vi "MCListManager.vi"(8 "error in (no error)":errorcluster, 9 "Path":path, 10 "Command":T1(ring), 11 "MCListbox Refnum":refnum<vi>) -> (0 "error out":errorcluster, 3 "MCListbox Refnum out":refnum<vi>)   [LabVIEW 2013, in "AnimatorXControl.xctl"]
uses:
  AnimatorXControl.xctl
panel:
  out "TempString":string
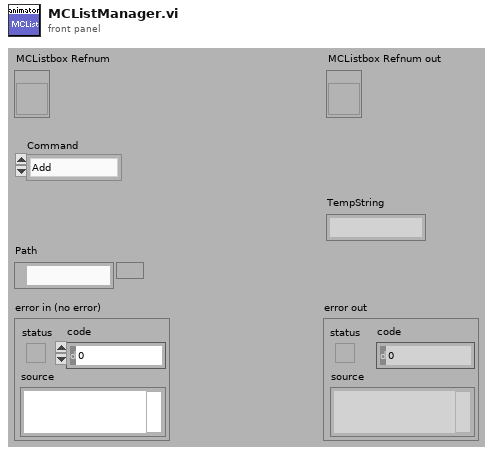
[diagram p1: front panel]
types:
  T1 = enum16{"Add", "Remove", "RemoveAll", "MoveUp", "MoveDown"}
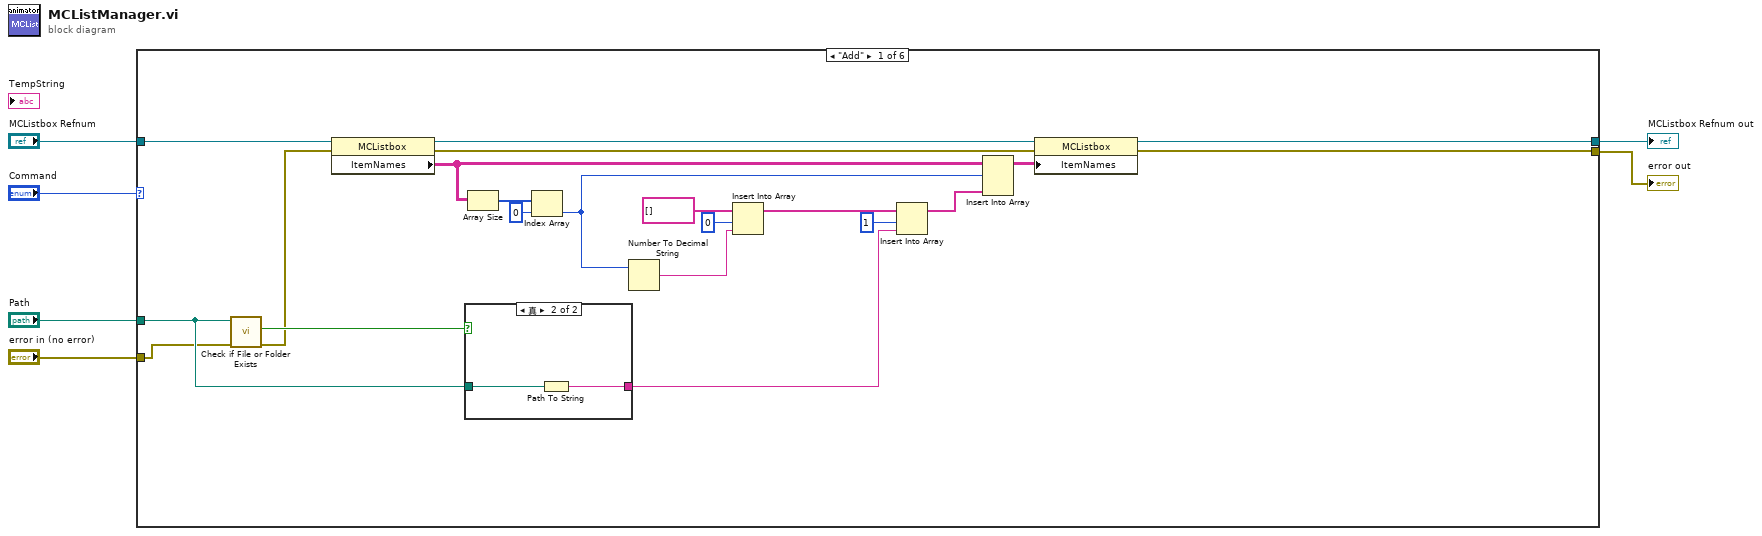
[diagram p0: block diagram]
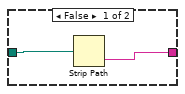
[diagram p2: hidden frame]
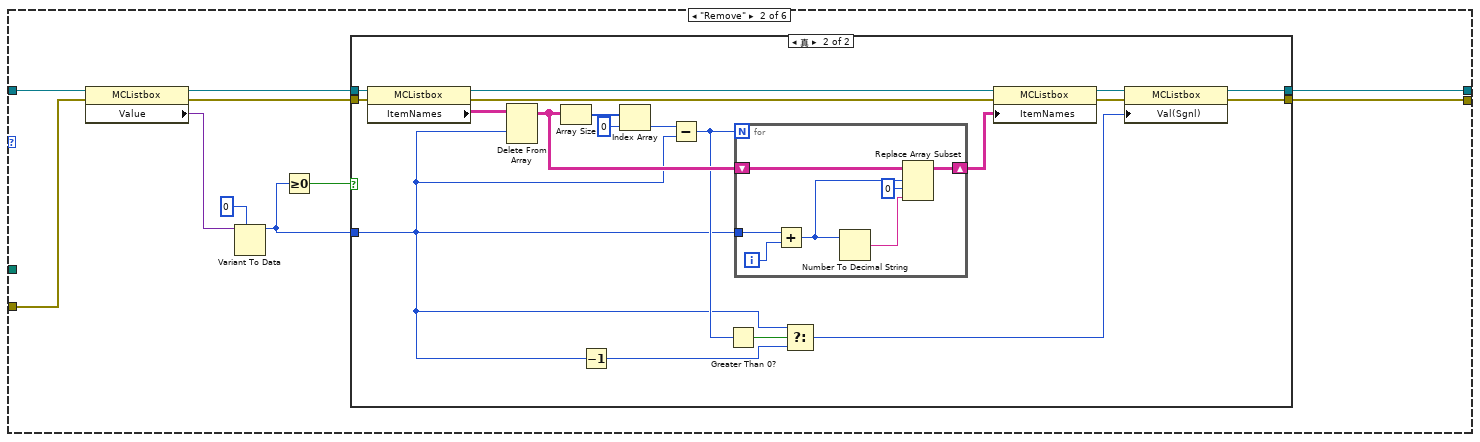
[diagram p3: hidden frame]
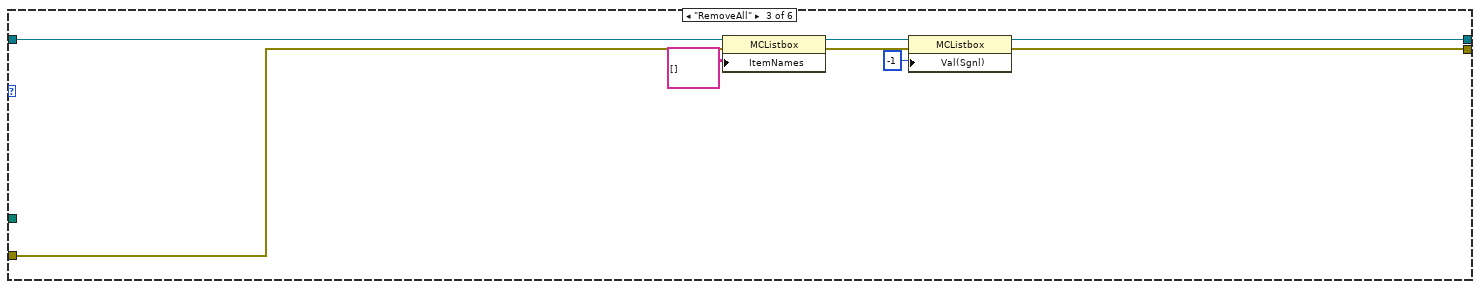
[diagram p5: hidden frame]
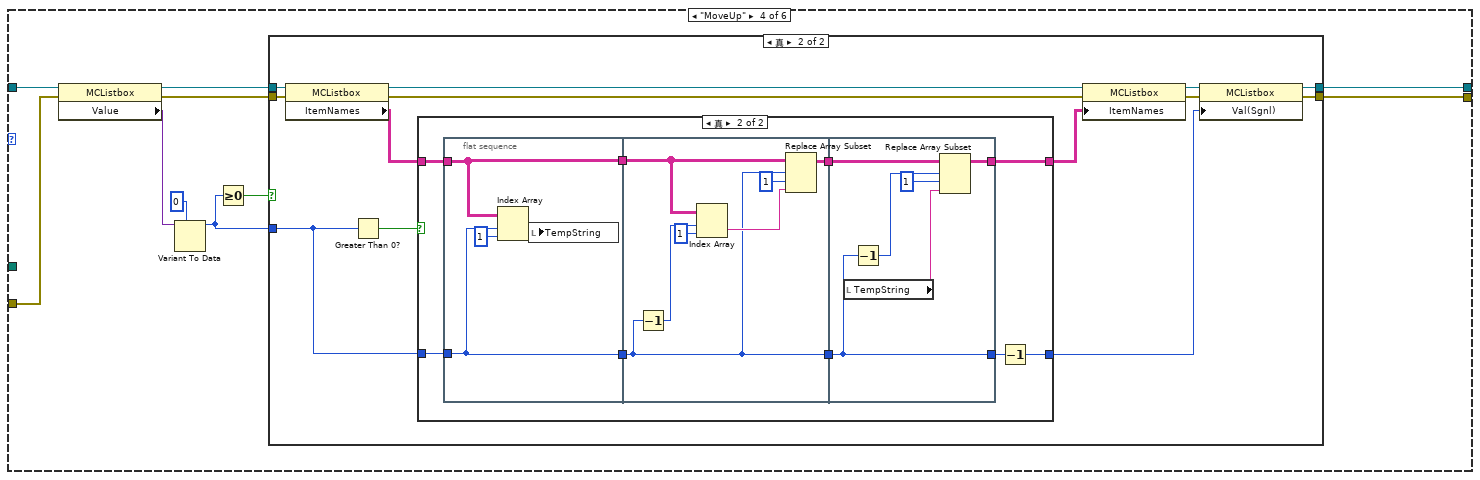
[diagram p6: hidden frame]
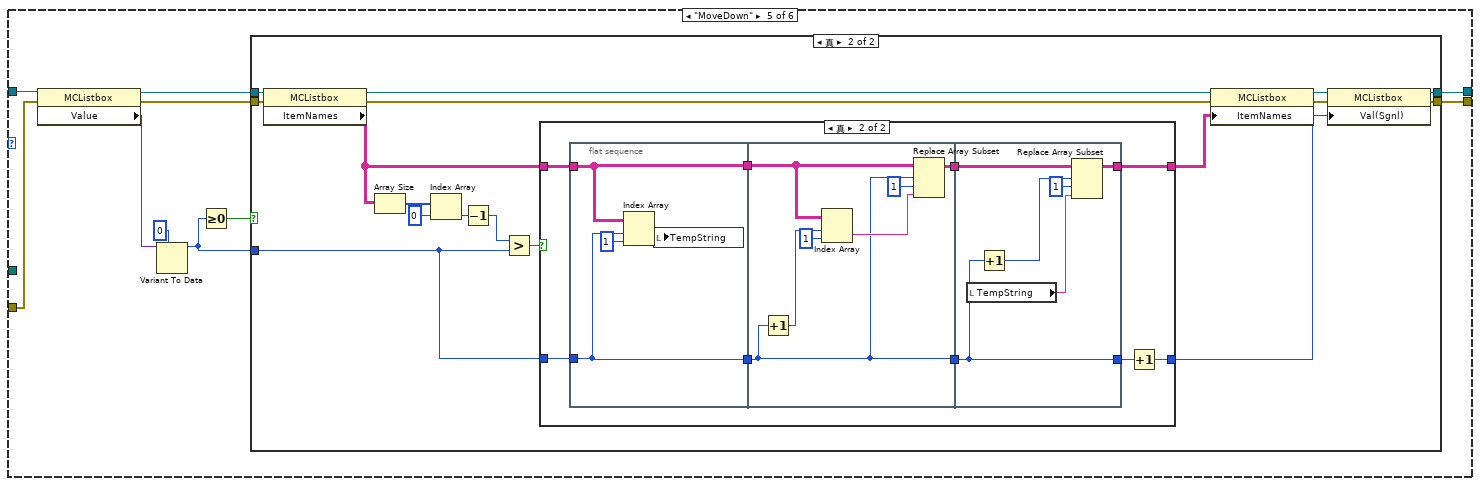
[diagram p9: hidden frame]
diagram:
  n1 = case shown="\"Add\"" "Command" {
    tunnel: "MCListbox Refnum" -> [w20 w36 w72 w87 w138 w188]
    tunnel: "Path" -> [w14 _ _ _ _ _]
    tunnel: [w9 w38 w73 w83 w137 w189] -> w3
    tunnel: "error in (no error)" -> [w11 w39 w71 w84 w136 w189]
    tunnel: [w8 w37 w74 w82 w135 w188] -> w1
    frame "Add" {
      n2 = call <vilib>:"Check if File or Folder Exists.vi"("error in (no error)"=w11, "path"=w14) -> ("error out"=w10:errorcluster, "file or folder exists?"=w15:bool)  [unwired: 7 in, 1 out]
      n3 = property class="MCListbox"(reference=w20, error in=w10) -> (reference out=w19:refnum<vi>, error out=w12:errorcluster, "ItemNames"=w22:string[][])
      n4 = case shown="真" w15 {
        tunnel: w14 -> [w29 w31]
        tunnel: [w28 w30] -> w13
        frame False {
          n5 = Strip Path(path=w29) -> (name=w28:string)  [unwired: 1 out]
        }
        frame True {
          n6 = Path To String(path=w31) -> (string=w30:string)
        }
      }
      n7 = Array Size(array=w22) -> (size(s)=w27:i32[])
      n8 = Index Array(array=w27, index=0) -> (element=w16:i32)
      n9 = Number To Decimal String(number=w16) -> (decimal integer string=w17:string)  [unwired: 1 in]
      n10 = Insert Into Array(array=string[] [], index=0 ("disabled index (col)"), new element=w17) -> (w7:string[])
      n11 = Insert Into Array(array=w7, index=1 ("disabled index (col)"), new element=w13) -> (w21:string[])
      n12 = Insert Into Array(array=w22, index (row)=w16, new element=w21) -> (w18:string[][])  [unwired: 1 in]
      n13 = property class="MCListbox"(reference=w19, error in=w12, "ItemNames"=w18) -> (reference out=w8:refnum<vi>, error out=w9:errorcluster)
    }
    frame "Remove" {
      n14 = property class="MCListbox"(reference=w36, error in=w39) -> (reference out=w41:refnum<vi>, error out=w40:errorcluster, "Value"=w35:variant)
      n15 = Variant To Data(type=0, Variant=w35) -> (data=w33:i32)  [unwired: 1 in, 1 out]
      n16 = Greater Or Equal To 0?(x=w33) -> (x >= 0?=w32:bool)
      n17 = case shown="真" w32 {
        tunnel: w41 -> [w43 w62]
        tunnel: w40 -> [w42 w61]
        tunnel: [w42 w47] -> w38
        tunnel: [w43 w46] -> w37
        tunnel: w33 -> [_ w44]
        frame False {
        }
        frame True {
          n18 = property class="MCListbox"(reference=w62, error in=w61) -> (reference out=w55:refnum<vi>, error out=w48:errorcluster, "ItemNames"=w60:string[][])
          n19 = Delete From Array(array=w60, index (row)=w44) -> (array with subset deleted=w56:string[][])  [unwired: 2 in, 1 out]
          n20 = Array Size(array=w56) -> (size(s)=w59:i32[])
          n21 = Decrement(x=w44) -> (x-1=w51:i32)
          n22 = Index Array(array=w59, index=0) -> (element=w57:i32)
          n23 = Subtract(x=w57, y=w44) -> (x-y=w53:i32)
          n24 = Greater Than 0?(x=w53) -> (x > 0?=w52:bool)
          n25 = for {
            N: w53 -> [_]
            shift-right: [w66] -> w54
            shift-left: w56 -> [w67]
            tunnel: w44 -> [w69]
            i -> [w68]
            n26 = Add(x=w69, y=w68) -> (x+y=w63:i32)
            n27 = Number To Decimal String(number=w63) -> (decimal integer string=w64:string)  [unwired: 1 in]
            n28 = Replace Array Subset(array=w67, new element=w64, index (row)=w63, index (col)=0 ("disabled index (col)")) -> (w66:string[][])
          }
          n29 = Select(t=w44, s=w52, f=w51) -> (s? t:f=w45:i32)
          n30 = property class="MCListbox"(reference=w55, error in=w48, "ItemNames"=w54) -> (reference out=w50:refnum<vi>, error out=w49:errorcluster)
          n31 = property class="MCListbox"(reference=w50, error in=w49, "Val(Sgnl)"=w45) -> (reference out=w46:refnum<vi>, error out=w47:errorcluster)
        }
      }
    }
    frame "RemoveAll" {
      n32 = property class="MCListbox"(reference=w72, error in=w71, "ItemNames"=string[][] [] ("Item Names")) -> (reference out=w77:refnum<vi>, error out=w75:errorcluster)
      n33 = property class="MCListbox"(reference=w77, error in=w75, "Val(Sgnl)"=-1) -> (reference out=w74:refnum<vi>, error out=w73:errorcluster)
    }
    frame "MoveUp" {
      n34 = property class="MCListbox"(reference=w87, error in=w84) -> (reference out=w86:refnum<vi>, error out=w85:errorcluster, "Value"=w81:variant)
      n35 = Variant To Data(type=0, Variant=w81) -> (data=w79:i32)  [unwired: 1 in, 1 out]
      n36 = Greater Or Equal To 0?(x=w79) -> (x >= 0?=w78:bool)
      n37 = case shown="真" w78 {
        tunnel: w86 -> [w89 w102]
        tunnel: w85 -> [w88 w101]
        tunnel: [w88 w94] -> w83
        tunnel: [w89 w93] -> w82
        tunnel: w79 -> [_ w91]
        frame False {
        }
        frame True {
          n38 = property class="MCListbox"(reference=w102, error in=w101) -> (reference out=w99:refnum<vi>, error out=w96:errorcluster, "ItemNames"=w100:string[][])
          n39 = Greater Than 0?(x=w91) -> (x > 0?=w90:bool)
          n40 = case shown="真" w90 {
            tunnel: w100 -> [w104 w113]
            tunnel: w91 -> [w103 w112]
            tunnel: [w104 w105] -> w98
            tunnel: [w103 w109] -> w92
            frame False {
            }
            frame True {
              n41 = flat-sequence {
                tunnel: w113 -> [w115]
                tunnel: w112 -> [w116]
                tunnel: [w116] -> w111
                tunnel: [w115] -> w108
                tunnel: w111 -> [w119]
                tunnel: w108 -> [w123]
                tunnel: [w119] -> w107
                tunnel: [w118] -> w106
                tunnel: [w128] -> w110
                tunnel: w107 -> [w128]
                tunnel: w106 -> [w129]
                tunnel: [w125] -> w105
                frame #0 {
                  n42 = Index Array(array=w115, index (row)=w116, index (col)=1 ("disabled index (col)")) -> (element=w114:string)
                  n43 = local write "TempString"(w114) -> ()
                }
                frame #1 {
                  n44 = Decrement(x=w119) -> (x-1=w122:i32)
                  n45 = Index Array(array=w123, index (row)=w122, index (col)=1 ("disabled index (col)")) -> (element=w121:string)
                  n46 = Replace Array Subset(array=w123, new element=w121, index (row)=w119, index (col)=1 ("disabled index (col)")) -> (w118:string[][])
                }
                frame #2 {
                  n47 = local read "TempString"() -> (w126:string)
                  n48 = Decrement(x=w128) -> (x-1=w127:i32)
                  n49 = Replace Array Subset(array=w129, new element=w126, index (row)=w127, index (col)=1 ("disabled index (col)")) -> (w125:string[][])
                }
              }
              n50 = Decrement(x=w110) -> (x-1=w109:i32)
            }
          }
          n51 = property class="MCListbox"(reference=w99, error in=w96, "ItemNames"=w98) -> (reference out=w97:refnum<vi>, error out=w95:errorcluster)
          n52 = property class="MCListbox"(reference=w97, error in=w95, "Val(Sgnl)"=w92) -> (reference out=w93:refnum<vi>, error out=w94:errorcluster)
        }
      }
    }
    frame "MoveDown" {
      n53 = property class="MCListbox"(reference=w138, error in=w136) -> (reference out=w140:refnum<vi>, error out=w139:errorcluster, "Value"=w134:variant)
      n54 = Variant To Data(type=0, Variant=w134) -> (data=w132:i32)  [unwired: 1 in, 1 out]
      n55 = Greater Or Equal To 0?(x=w132) -> (x >= 0?=w131:bool)
      n56 = case shown="真" w131 {
        tunnel: w140 -> [w142 w159]
        tunnel: w139 -> [w141 w158]
        tunnel: [w141 w146] -> w137
        tunnel: [w142 w145] -> w135
        tunnel: w132 -> [_ w143]
        frame False {
        }
        frame True {
          n57 = property class="MCListbox"(reference=w159, error in=w158) -> (reference out=w154:refnum<vi>, error out=w151:errorcluster, "ItemNames"=w155:string[][])
          n58 = Array Size(array=w155) -> (size(s)=w157:i32[])
          n59 = Index Array(array=w157, index=0) -> (element=w149:i32)
          n60 = Decrement(x=w149) -> (x-1=w147:i32)
          n61 = Greater?(x=w147, y=w143) -> (0:w148:bool)
          n62 = case shown="真" w148 {
            tunnel: w155 -> [w161 w165]
            tunnel: w143 -> [w160 w164]
            tunnel: [w161 w163] -> w153
            tunnel: [w160 w170] -> w144
            frame False {
            }
            frame True {
              n63 = flat-sequence {
                tunnel: w165 -> [w172]
                tunnel: w164 -> [w173]
                tunnel: [w173] -> w169
                tunnel: [w172] -> w168
                tunnel: w169 -> [w176]
                tunnel: w168 -> [w180]
                tunnel: [w176] -> w167
                tunnel: [w175] -> w166
                tunnel: [w185] -> w162
                tunnel: w167 -> [w185]
                tunnel: w166 -> [w186]
                tunnel: [w183] -> w163
                frame #0 {
                  n64 = Index Array(array=w172, index (row)=w173, index (col)=1 ("disabled index (col)")) -> (element=w171:string)
                  n65 = local write "TempString"(w171) -> ()
                }
                frame #1 {
                  n66 = Increment(x=w176) -> (x+1=w179:i32)
                  n67 = Index Array(array=w180, index (row)=w179, index (col)=1 ("disabled index (col)")) -> (element=w178:string)
                  n68 = Replace Array Subset(array=w180, new element=w178, index (row)=w176, index (col)=1 ("disabled index (col)")) -> (w175:string[][])
                }
                frame #2 {
                  n69 = local read "TempString"() -> (w182:string)
                  n70 = Increment(x=w185) -> (x+1=w184:i32)
                  n71 = Replace Array Subset(array=w186, new element=w182, index (row)=w184, index (col)=1 ("disabled index (col)")) -> (w183:string[][])
                }
              }
              n72 = Increment(x=w162) -> (x+1=w170:i32)
            }
          }
          n73 = property class="MCListbox"(reference=w154, error in=w151, "ItemNames"=w153) -> (reference out=w152:refnum<vi>, error out=w150:errorcluster)
          n74 = property class="MCListbox"(reference=w152, error in=w150, "Val(Sgnl)"=w144) -> (reference out=w145:refnum<vi>, error out=w146:errorcluster)
        }
      }
    }
    frame Default {
    }
  }
  "error out" <- w3
  "MCListbox Refnum out" <- w1
